vi "trial stroke report code.vi"() -> ()   [LabVIEW 2025]
panel:
  out "error out":errorcluster
  out "return value":string
  in  "footer_link_url":string="https://www.paltro.com/products/product-selector/lubricity"
  in  "logo_path":path=path "C:/LAB-IQ/lib/paltro logo.png"
  in  "logo_link_url":string="https://www.paltro.com/"
  in  "output_dir":path=path "C:/LAB-IQ/Data/Stroke Calibration"
  in  "measured_value":dbl
  in  "operator_name":string="Kiran"
  in  "Instrument_serial Number":string="021099"
  in  "error in (no error)":errorcluster
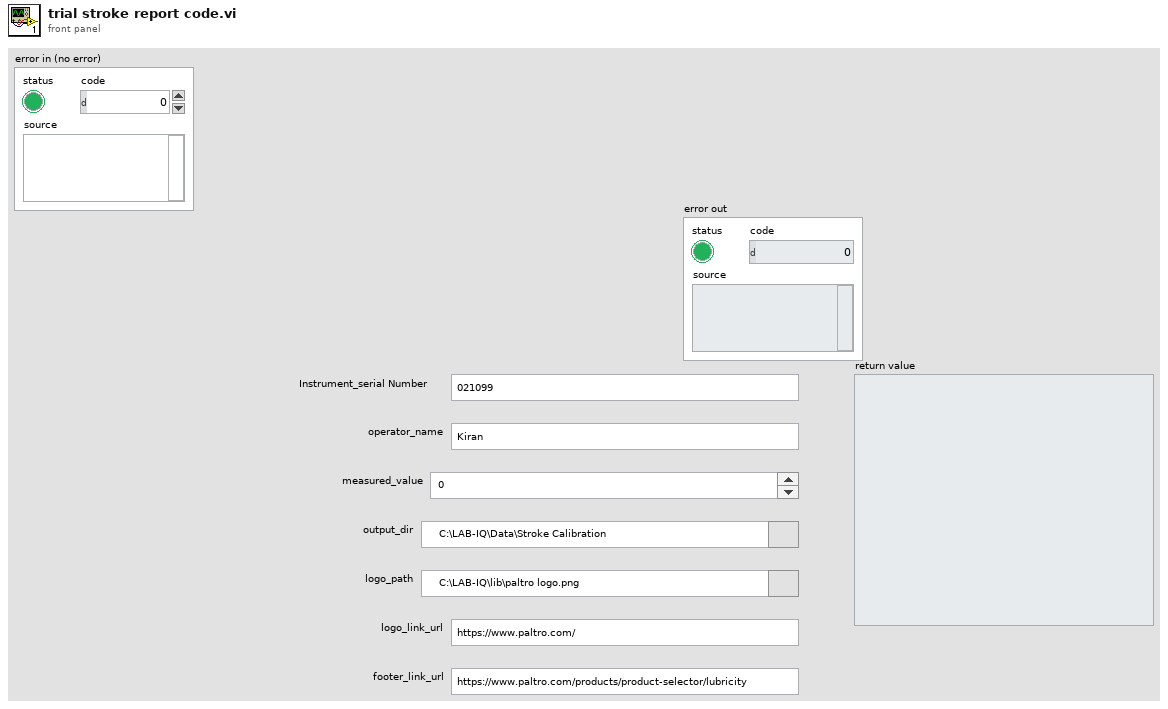
[diagram p1: front panel]
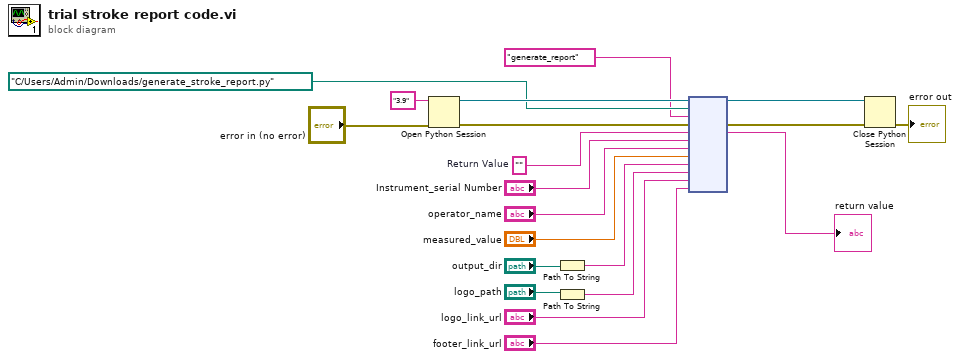
[diagram p0: block diagram]
diagram:
  w14 = ""  # Return Value
  n1 = Open Python Session(python version="3.9" ("Python version"), 3:"error in (no error)") -> (session out=w19:refnum<k35>, error out=w17:errorcluster)  [unwired: 1 in]
  n2 = Path To String(path="output_dir") -> (string=w8:string)
  n3 = Path To String(path="logo_path") -> (string=w7:string)
  n4 = node(w19, path "C:/Users/Admin/Downloads/generate_stroke_report.py" ("Python path"), "generate_report" ("function name"), w17, w14, "Instrument_serial Number", "operator_name", "measured_value", w8, w7, "logo_link_url", "footer_link_url") -> (w2:refnum<k35>, w3:errorcluster, →"return value":string)  [unwired: 7 in, 2 out]
  n5 = Close Python Session(session in=w2, error in=w3) -> (11:→"error out":errorcluster)
